vi "Check For Abort.vi"(2 "Mixed Mode State In":T5, 3 "Within Limits":T1[](array[typedef])) -> (0 "Faulted":bool, 1 "Mixed Mode State Out":T5)   [LabVIEW 2009]
uses:
  MixedMode/Mixed Mode States.ctl
  Limits/Within Limits Matrix.ctl
  Limits/Actuator Faults.ctl
  Limits/Cart Disp Faults.ctl
  Limits/Cart Force Faults.ctl
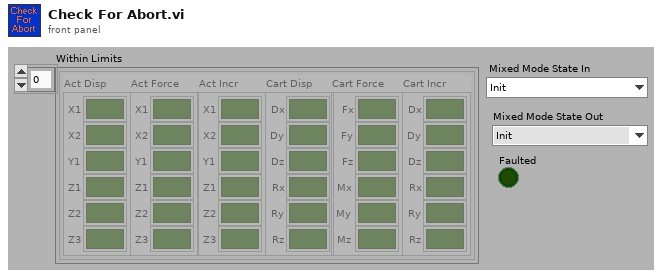
[diagram p1: front panel]
types:
  T1 = typedef "Within Limits Matrix.ctl" = cluster{"Act Disp":T2, "Act Force":T2, "Act Incr":T2, "Cart Disp":T3, "Cart Force":T4, "Cart Incr":T3}
  T2 = typedef "Actuator Faults.ctl" = cluster{"X1":bool, "X2":bool, "Y1":bool, "Z1":bool, "Z2":bool, "Z3":bool}
  T3 = typedef "Cart Disp Faults.ctl" = cluster{"Dx":bool, "Dy":bool, "Dz":bool, "Rx":bool, "Ry":bool, "Rz":bool}
  T4 = typedef "Cart Force Faults.ctl" = cluster{"Fx":bool, "Fy":bool, "Fz":bool, "Mx":bool, "My":bool, "Mz":bool}
  T5 = typedef "Mixed Mode States.ctl" = enum16{"Init", "Wait For DAQ", "Idle", "Start Initial Position", "Initial Position", "Start Initial Ramp", "Run Initial Ramp", "Start Iterative Stage", "Convergence Check", "Update Stiffness Jacobian", "Update Command", "Start Iterative Ramp", "Run Iterative Ramp", "Start Iterative Stabilize", "Iterative Stabilize", "Start Iterative Holding", "Iterative Holding", "Start Stabilize", "Stabilize", "Start Hold", "Holding", "Done", "Aborting", "Exit", "Nop"}
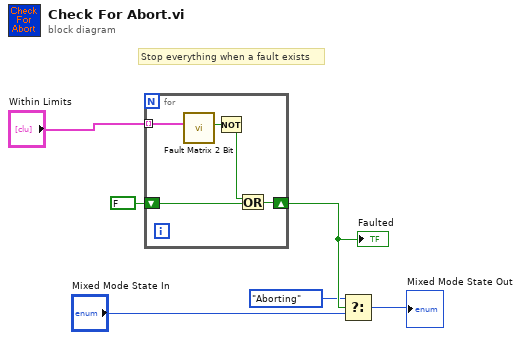
[diagram p0: block diagram]
diagram:
  # "Stop everything when a fault exists"
  n1 = for {
    tunnel: "Within Limits" -> [w11] mode=indexing
    shift-right: [w9] -> w6
    shift-left: FALSE -> [w7]
    n2 = call "Fault Matrix 2 Bit.vi"("Within Limits"=w11) -> ("No Faults"=w10:bool)  [unwired: 10 out]
    n3 = Not(x=w10) -> (.not. x?=w8:bool)
    n4 = Or(x=w8, y=w7) -> (x .or. y?=w9:bool)
  }
  "Faulted" <- w6
  n5 = Select(t=Mixed_Mode_States."Aborting", s=w6, f="Mixed Mode State In") -> (s? t:f=→"Mixed Mode State Out":T5)
